vi "Teleop.vi"(10 "Match Info":T1={"Autonomous Elapsed Seconds"=0.0, "TeleOp Elapsed Seconds"=0.0, "Disabled Elapsed Seconds"=0.0, "Visited Autonomous"=FALSE, "Visited TeleOp"=FALSE, "Visited Disabled"=FALSE, "Autonomous Settings"={"Autonomous Style"=enum."Independent", "VI Refnum"=refnum}}, 11 "Call Context":T2) -> ()   [LabVIEW 2018]
doc: "This VI is called for each TeleOp packet received from the DS where the robot is not disabled. It is often used to read from the joysticks and update I/O or to update setpoints for timed control loops. It should complete and return within 20 milliseconds or it may miss DS packets."
uses:
  <vilib>/Rock Robotics/WPI/DriverStation/WPI_DriverStationDerivedRobotMode.ctl
  <vilib>/Rock Robotics/WPI/DriverStation/WPI_DriverStationMatch Info.ctl
  <vilib>/Rock Robotics/WPI/Solenoid/WPI_SolenoidValue.ctl
  <vilib>/Rock Robotics/WPI/ThirdParty/Phoenix-LabVIEW/Motor Controller/Controls/CTRE_Phoenix_MotorControl_ControlMode.ctl
  <vilib>/Rock Robotics/WPI/Utilities/WPI_GetSetVariantRefNum.vi
  Robot Global Data.vi
  <vilib>/Rock Robotics/Network Tables/NT Write Boolean Array.vi
  <vilib>/Rock Robotics/Network Tables/NT Write Numeric Array.vi
  <vilib>/Rock Robotics/Network Tables/NT Read Boolean.vi
  <vilib>/Rock Robotics/Network Tables/NT Read Number.vi
  <vilib>/Rock Robotics/WPI/Solenoid/WPI_SolenoidSetEnum.vi
panel:
  out "Sample Slider 0":dbl(slide) scale=0.0..5.0
  out "Sample Boolean 1":bool
  out "Sample Boolean 0":bool
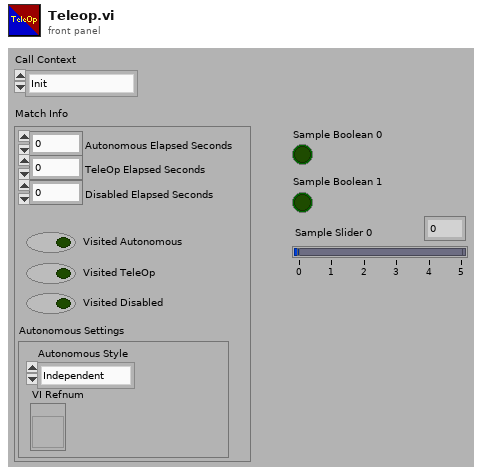
[diagram p1: front panel]
types:
  T1 = typedef "WPI_DriverStationMatch Info.ctl" = cluster{"Autonomous Elapsed Seconds":dbl, "TeleOp Elapsed Seconds":dbl, "Disabled Elapsed Seconds":dbl, "Visited Autonomous":bool, "Visited TeleOp":bool, "Visited Disabled":bool, "Autonomous Settings":cluster{"Autonomous Style":enum16{"Iterative", "Independent"}, "VI Refnum":refnum<vi>}}
  T2 = typedef "WPI_DriverStationDerivedRobotMode.ctl" = enum16{"Init", "Execute", "Stop"}
  T3 = typedef "CTRE_Phoenix_MotorControl_ControlMode.ctl" = u16
  T4 = typedef "WPI_SolenoidValue.ctl" = enum16{"Off", "On", "Forward", "Reverse"}
  T5 = typedef "WPI_JoystickDevRef.ctl" = cluster{"Device":T6}
  T6 = typedef "WPI_JoystickDeviceEnum.ctl" = enum16{"USB 0", "USB 1", "USB 2", "USB 3", "USB 4", "USB 5"}
  T7 = typedef "WPI_RobotDriveDevRef.ctl" = cluster{"DevStatus":errorcluster, "Motors[]":T8[], "Square Inputs":bool, "Max Output":dbl}
  T8 = typedef "WPI_MotorControlDeviceRef.ctl" = cluster{"DeviceStatus":errorcluster, "Type":T9, "PWM":cluster{"PWM Channel":T10, "DeadBand":T11}, "CAN":cluster{"Device Number":u8, "SetOutput VI Ref":variant, "GetOutput VI Ref":variant, "Enable VI Ref":variant, "Disable VI Ref":variant, "Data":variant}, "Invert":bool, "DIO PWM":cluster{"PWM \"Enable\" Channel":T10, "DIOChannel":T12, "PWM Rate":dbl}}
  T9 = typedef "WPI_MotorControlType.ctl" = enum16{"PWM", "CAN", "DIO PWM"}
  T10 = typedef "FPGA_DIOPWMChannel.ctl" = enum8{"PWM 0", "PWM 1", "PWM 2", "PWM 3", "PWM 4", "PWM 5", "PWM 6", "PWM 7", "PWM 8", "PWM 9", "PWM MXP 0", "PWM MXP 1", "PWM MXP 2", "PWM MXP 3", "PWM MXP 4", "PWM MXP 5", "PWM MXP 6", "PWM MXP 7", "PWM MXP 8", "PWM MXP 9", "Invalid"}
  T11 = typedef "WPI_PWMDeadband.ctl" = cluster{"Name":string, "maxPositivePwm":i32, "minPositivePwm":i32, "centerPwm":i32, "maxNegativePwm":i32, "minNegativePwm":i32, "angularRange":u16}
  T12 = typedef "FPGA_DIOChannel.ctl" = enum8{"DIO 0", "DIO 1", "DIO 2", "DIO 3", "DIO 4", "DIO 5", "DIO 6", "DIO 7", "DIO 8", "DIO 9", "DIO MXP 0", "DIO MXP 1", "DIO MXP 2", "DIO MXP 3", "DIO MXP 4", "DIO MXP 5", "DIO MXP 6", "DIO MXP 7", "DIO MXP 8", "DIO MXP 9", "DIO MXP 10", "DIO MXP 11", "DIO MXP 12", "DIO MXP 13", "DIO MXP 14", "DIO MXP 15", "SPI Port CS1", "SPI Port CS2", "SPI Port CS3", "SPI Port MISO", "SPI Port MOSI", "Invalid"}
  T13 = cluster{"Buttons[0]":bool, "Buttons[1]":bool, "Buttons[2]":bool, "Buttons[3]":bool, "Buttons[4]":bool, "Buttons[5]":bool, "Buttons[6]":bool, "Buttons[7]":bool, "Buttons[8]":bool, "Buttons[9]":bool, "Buttons[10]":bool}
  T14 = typedef "WPI_SolenoidDevRef.ctl" = cluster{"DevStatus":errorcluster, "Pneumatics Control Module":u8, "Forward Solenoid Channel":T15, "Reverse Solenoid Channel":T15}
  T15 = typedef "WPI_SolenoidChannel.ctl" = enum8{"Solenoid 0", "Solenoid 1", "Solenoid 2", "Solenoid 3", "Solenoid 4", "Solenoid 5", "Solenoid 6", "Solenoid 7", "Invalid"}
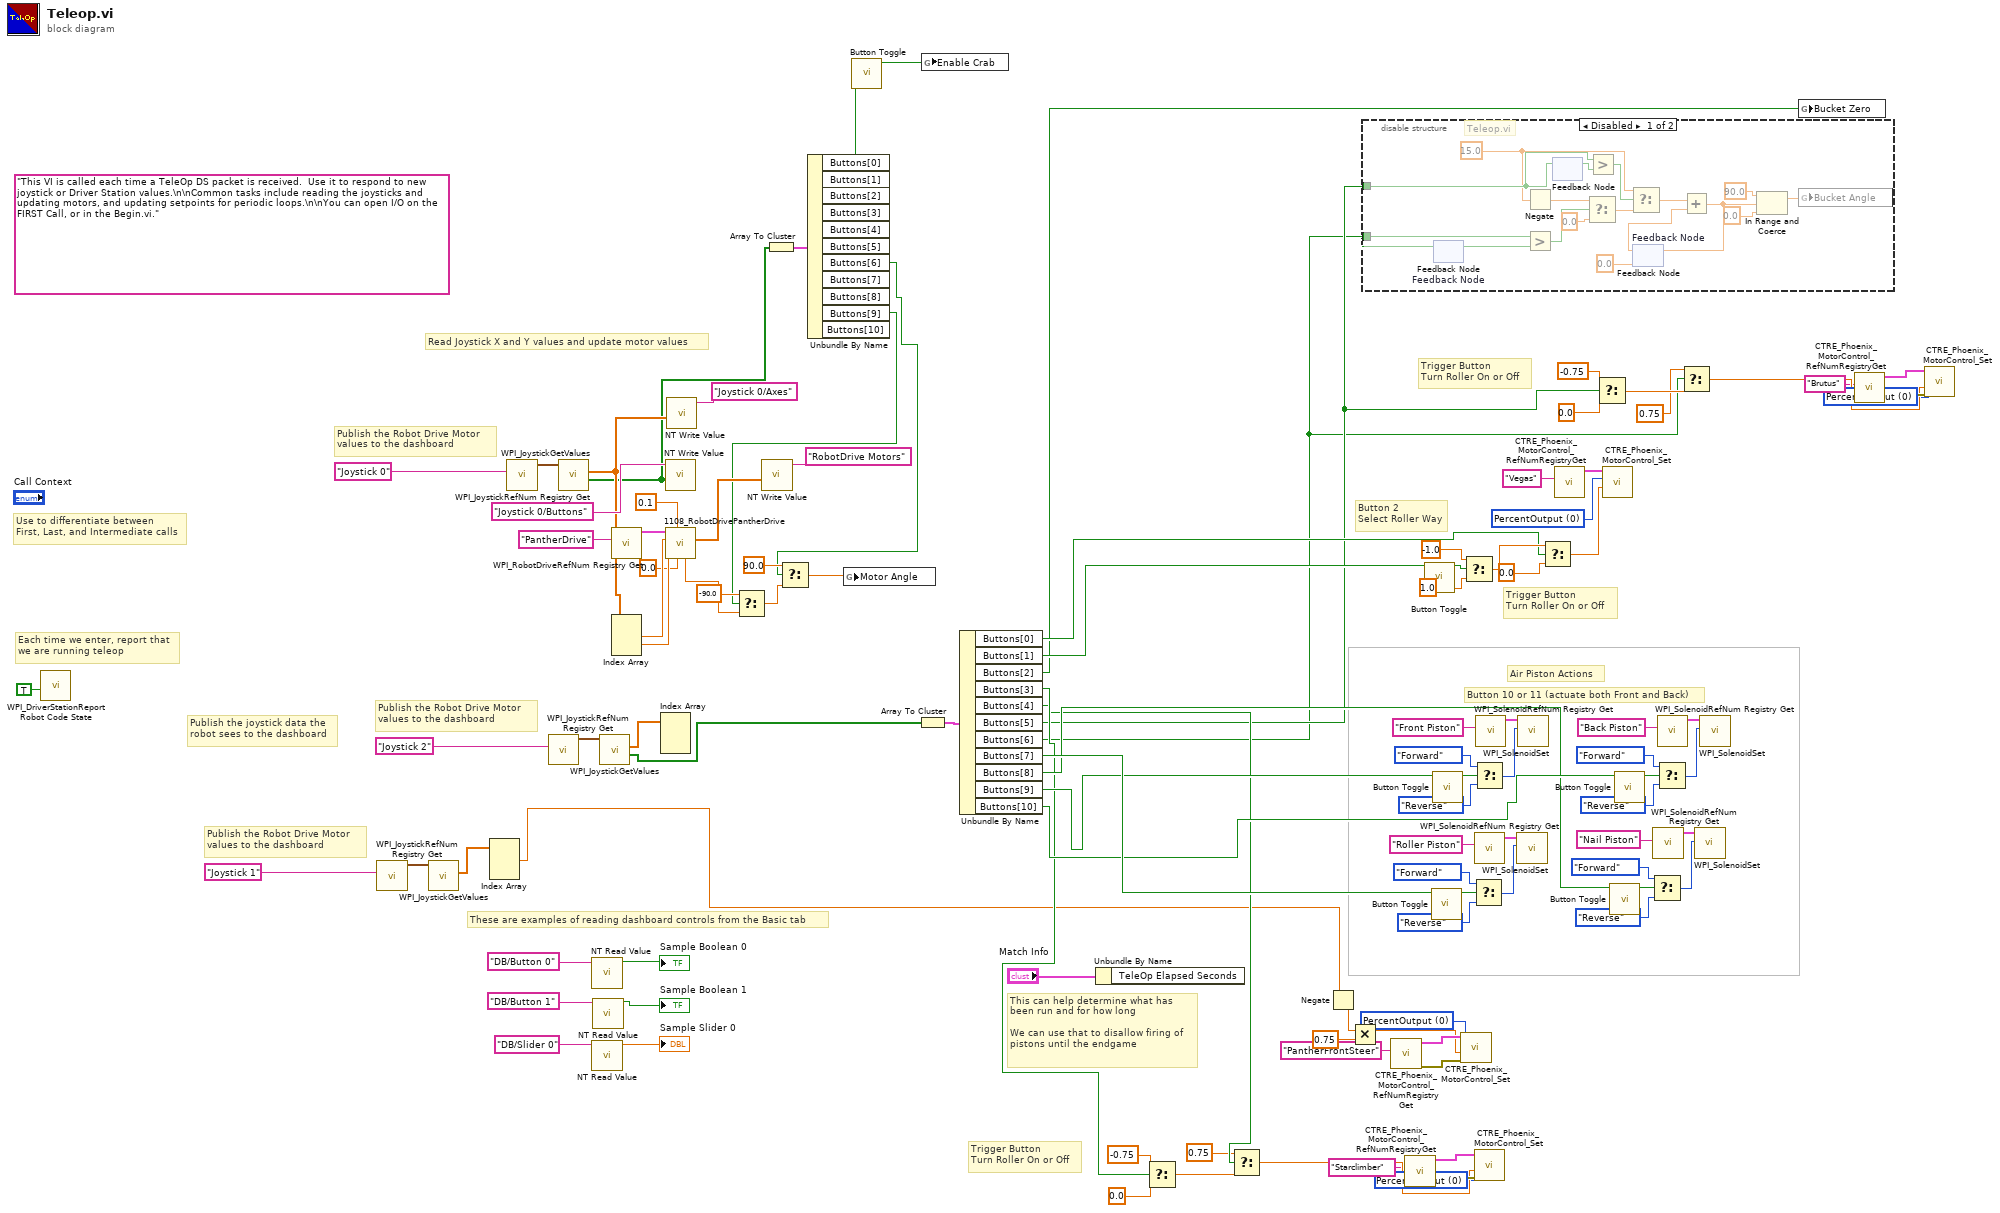
[diagram p0: block diagram]
diagram:
  w23 = T3 0 items=["PercentOutput"=0, "Position"=1, "Velocity"=2, "Current"=3, "Follower"=5, "MotionProfile"=6, "MotionMagic"=7, "MotionProfileArc"=10, "Disabled"=15] ("Control Mode")
  w32 = T3 0 items=["PercentOutput"=0, "Position"=1, "Velocity"=2, "Current"=3, "Follower"=5, "MotionProfile"=6, "MotionMagic"=7, "MotionProfileArc"=10, "Disabled"=15] ("Control Mode")
  w43 = T3 0 items=["PercentOutput"=0, "Position"=1, "Velocity"=2, "Current"=3, "Follower"=5, "MotionProfile"=6, "MotionMagic"=7, "MotionProfileArc"=10, "Disabled"=15] ("Control Mode")
  w59 = T3 0 items=["PercentOutput"=0, "Position"=1, "Velocity"=2, "Current"=3, "Follower"=5, "MotionProfile"=6, "MotionMagic"=7, "MotionProfileArc"=10, "Disabled"=15] ("Control Mode")
  (unwired) "This VI is called each time a TeleOp DS packet is received.  Use it to respond to new joystick or Driver Station values.\n\nCommon tasks include reading the joysticks and updating motors, and updating setpoints for periodic loops.\n\nYou can open I/O on the FIRST Call, or in the Begin.vi."
  # "Publish the Robot Drive Motor\nvalues to the dashboard"
  # "Trigger Button\nTurn Roller On or Off"
  # "Trigger Button\nTurn Roller On or Off"
  # "Button 2\nSelect Roller Way"
  # "Trigger Button\nTurn Roller On or Off"
  # "Button 10 or 11 (actuate both Front and Back)"
  # "Air Piston Actions"
  # "Publish the Robot Drive Motor\nvalues to the dashboard"
  # "These are examples of reading dashboard controls from the Basic tab"
  # "Publish the Robot Drive Motor\nvalues to the dashboard"
  # "Publish the joystick data the\nrobot sees to the dashboard"
  # "Each time we enter, report that\nwe are running teleop"
  # "Use to differentiate between\nFirst, Last, and Intermediate calls"
  # "This can help determine what has\nbeen run and for how long\n\nWe can use that to disallow firing of\npistons until the endgame"
  # "Read Joystick X and Y values and update motor values"
  n1 = call <vilib>:"WPI_DriverStationReport Robot Code State.vi"("TeleOp"=TRUE ("Autonomous")) -> ()  [unwired: 10 in, 1 out]
  n2 = call <vilib>:"WPI_JoystickRefNum Registry Get.vi"("refnum name"="Joystick 1") -> ("JoystickDevRef"=w15:T5)  [unwired: 1 in, 9 out]
  n3 = call <vilib>:"WPI_JoystickGetValues.vi"("JoystickDevRef"=w15) -> ("Axes"=w14:dbl[])  [unwired: 6 in, 4 out]
  n4 = Index Array(array=w14) -> (element #1=w13:dbl)  [unwired: 3 in, 2 out]
  n5 = call <vilib>:"WPI_JoystickRefNum Registry Get.vi"("refnum name"="Joystick 0") -> ("JoystickDevRef"=w107:T5)  [unwired: 1 in, 9 out]
  n6 = call <vilib>:"WPI_JoystickRefNum Registry Get.vi"("refnum name"="Joystick 2") -> ("JoystickDevRef"=w90:T5)  [unwired: 1 in, 9 out]
  n7 = call <vilib>:"WPI_JoystickGetValues.vi"("JoystickDevRef"=w107) -> ("Buttons"=w11:bool[], "Axes"=w103:dbl[])  [unwired: 6 in, 3 out]
  n8 = call-poly <vilib>:"NT Read Value.vi"("Name"="DB/Button 0" ("refnum name")) -> ("Boolean"=→"Sample Boolean 0":bool)  [unwired: 9 in, 1 out]
  n9 = call-poly <vilib>:"NT Read Value.vi"("Name"="DB/Slider 0" ("refnum name")) -> ("Numeric"=→"Sample Slider 0":dbl)  [unwired: 9 in, 1 out]
  n10 = call-poly <vilib>:"NT Read Value.vi"("Name"="DB/Button 1" ("refnum name")) -> ("Boolean"=→"Sample Boolean 1":bool)  [unwired: 9 in, 1 out]
  n11 = call <vilib>:"WPI_JoystickGetValues.vi"("JoystickDevRef"=w90) -> ("Buttons"=w87:bool[], "Axes"=w89:dbl[])  [unwired: 6 in, 3 out]
  n12 = call <vilib>:"WPI_RobotDriveRefNum Registry Get.vi"("refnum name"="PantherDrive") -> ("RobotDriveDevRef"=w94:T7)  [unwired: 1 in, 9 out]
  n13 = Index Array(array=w103) -> (element #1=w93:dbl, element #2=w92:dbl)  [unwired: 3 in, 1 out]
  n14 = Index Array(array=w89) -> ()  [unwired: 3 in, 3 out]
  n15 = call-poly <vilib>:"NT Write Value.vi"("Boolean Array"=w11, "Name"="Joystick 0/Buttons") -> ()  [unwired: 9 in, 1 out]
  n16 = call "1108_RobotDrivePantherDrive.vi"("x-spin"=0.0, "Deadband"=0.1, "y"=w92, "x"=w93, "RobotDriveDevRef"=w94) -> ("Motor Values"=w95:dbl[], "Motor angle"=w8:dbl)  [unwired: 3 in, 2 out]
  n17 = call-poly <vilib>:"NT Write Value.vi"("Numeric Array"=w103, "Name"="Joystick 0/Axes") -> ()  [unwired: 9 in, 1 out]
  n18 = call-poly <vilib>:"NT Write Value.vi"("Numeric Array"=w95, "Name"="RobotDrive Motors") -> ()  [unwired: 9 in, 1 out]
  n19 = Array To Cluster(array=w11) -> (cluster=w12:T13)
  n20 = Unbundle By Name(w12) -> ("Buttons[0]"=w10:bool, "Buttons[6]"=w3:bool, "Buttons[9]"=w4:bool)  [unwired: 8 out]
  n21 = Select(t=-90.0, s=w4, f=w8) -> (s? t:f=w7:dbl)
  n22 = Select(t=90.0, s=w3, f=w7) -> (s? t:f=w2:dbl)
  n23 = global write "Robot Global Data.vi" "Motor Angle"(w2) -> ()
  n24 = call "Button Toggle.vi"("Button Input"=w10) -> ("Toggled Output"=w9:bool)  [unwired: 10 in]
  n25 = Array To Cluster(array=w87) -> (cluster=w88:T13)
  n26 = global write "Robot Global Data.vi" "Enable Crab"(w9) -> ()
  n27 = Unbundle By Name(w88) -> ("Buttons[0]"=w51:bool, "Buttons[1]"=w55:bool, "Buttons[2]"=w50:bool, "Buttons[3]"=w36:bool, "Buttons[4]"=w35:bool, "Buttons[5]"=w20:bool, "Buttons[6]"=w19:bool, "Buttons[7]"=w52:bool, "Buttons[8]"=w42:bool, "Buttons[9]"=w48:bool, "Buttons[10]"=w49:bool)
  n28 = Unbundle By Name("Match Info") -> ()  [unwired: 1 out]
  n29 = Select(t=-0.75, s=w36, f=0.0) -> (s? t:f=w31:dbl)
  n30 = Select(t=0.75 ("f"), s=w35, f=w31) -> (s? t:f=w37:dbl)
  n31 = Negate(x=w13) -> (-x=w17:dbl)
  n32 = Multiply(x=w17, y=0.75) -> (x*y=w45:dbl)
  n33 = disable-structure shown="Disabled" {
    disable-tunnel: w19 -> [w118 _]
    disable-tunnel: w20 -> [w117 _]
    frame Disabled {
      w115 = 15.0 ("t")
      # "Teleop.vi"
      n34 = feedback #1 "Feedback Node"() -> (w126:bool)  [unwired: 1 in]
      n35 = feedback-in #1(w118) -> ()
      n36 = Negate(x=w115) -> (-x=w114:dbl)
      n37 = Greater?(x=w118, y=w126) -> (0:w125:bool)
      n38 = feedback #2() -> (w127:bool)  [unwired: 1 in]
      n39 = feedback-in #2(w117) -> ()
      n40 = Select(t=w114, s=w125, f=0.0) -> (s? t:f=w123:dbl)
      n41 = Greater?(x=w117, y=w127) -> (0:w122:bool)
      n42 = Select(t=w115, s=w122, f=w123) -> (s? t:f=w121:dbl)
      n43 = feedback #3 "Feedback Node"(0.0) -> (w120:dbl)
      n44 = Add(x=w121, y=w120) -> (x+y=w116:dbl)
      n45 = feedback-in #3(w116) -> ()
      n46 = In Range and Coerce(upper limit=90.0, x=w116, lower limit=0.0) -> (coerced(x)=w111:dbl)  [unwired: 1 out]
      n47 = global write "Robot Global Data.vi" "Bucket Angle"(w111) -> ()
    }
    frame Enabled {
    }
  }
  n48 = call <vilib>:"CTRE_Phoenix_MotorControl_RefNumRegistryGet.vi"("refnum name"="PantherFrontSteer") -> ("error out"=w47:errorcluster, "PhoenixMotorControlDevRef"=w46:T8)  [unwired: 9 in]
  n49 = call <vilib>:"CTRE_Phoenix_MotorControl_RefNumRegistryGet.vi"("refnum name"="Starclimber") -> ("error out"=w41:errorcluster, "PhoenixMotorControlDevRef"=w40:T8)  [unwired: 9 in]
  n50 = call "Button Toggle.vi"("Button Input"=w55) -> ("Toggled Output"=w62:bool)  [unwired: 10 in]
  n51 = call "Button Toggle.vi"("Button Input"=w52) -> ("Toggled Output"=w74:bool)  [unwired: 10 in]
  n52 = call "Button Toggle.vi"("Button Input"=w48) -> ("Toggled Output"=w86:bool)  [unwired: 10 in]
  n53 = call <vilib>:"CTRE_Phoenix_MotorControl_Set.vi"("error in (no error)"=w47, "Output"=w45, "Control Mode"=w43, "PhoenixMotorControlDevRef"=w46) -> ()  [unwired: 6 in, 2 out]
  n54 = Select(t=-1.0, s=w62, f=1.0) -> (s? t:f=w56:dbl)
  n55 = Select(t=WPI_SolenoidValue."Forward" ("Value"), s=w74, f=WPI_SolenoidValue."Reverse" ("Value")) -> (s? t:f=w73:T4)
  n56 = Select(t=WPI_SolenoidValue."Forward" ("Value"), s=w86, f=WPI_SolenoidValue."Reverse" ("Value")) -> (s? t:f=w85:T4)
  n57 = call <vilib>:"WPI_SolenoidRefNum Registry Get.vi"("refnum name"="Roller Piston") -> ("SolenoidDevRef"=w70:T14)  [unwired: 9 in, 1 out]
  n58 = call <vilib>:"CTRE_Phoenix_MotorControl_Set.vi"("error in (no error)"=w41, "Output"=w37, "Control Mode"=w32, "PhoenixMotorControlDevRef"=w40) -> ()  [unwired: 6 in, 2 out]
  n59 = call <vilib>:"WPI_SolenoidRefNum Registry Get.vi"("refnum name"="Front Piston") -> ("SolenoidDevRef"=w82:T14)  [unwired: 9 in, 1 out]
  n60 = call-poly <vilib>:"WPI_SolenoidSet.vi"("Value"=w73, "SolenoidDevRef"=w70) -> ()  [unwired: 8 in, 2 out]
  n61 = call-poly <vilib>:"WPI_SolenoidSet.vi"("Value"=w85, "SolenoidDevRef"=w82) -> ()  [unwired: 8 in, 2 out]
  n62 = Select(t=w56, s=w51, f=0.0) -> (s? t:f=w53:dbl)
  n63 = call <vilib>:"CTRE_Phoenix_MotorControl_RefNumRegistryGet.vi"("refnum name"="Vegas") -> ("PhoenixMotorControlDevRef"=w61:T8)  [unwired: 9 in, 1 out]
  n64 = Select(t=-0.75, s=w20, f=0.0) -> (s? t:f=w22:dbl)
  n65 = call <vilib>:"CTRE_Phoenix_MotorControl_Set.vi"("Output"=w53, "Control Mode"=w59, "PhoenixMotorControlDevRef"=w61) -> ()  [unwired: 7 in, 2 out]
  n66 = call "Button Toggle.vi"("Button Input"=w42) -> ("Toggled Output"=w68:bool)  [unwired: 10 in]
  n67 = call "Button Toggle.vi"("Button Input"=w49) -> ("Toggled Output"=w80:bool)  [unwired: 10 in]
  n68 = Select(t=WPI_SolenoidValue."Forward" ("Value"), s=w68, f=WPI_SolenoidValue."Reverse" ("Value")) -> (s? t:f=w67:T4)
  n69 = call <vilib>:"WPI_SolenoidRefNum Registry Get.vi"("refnum name"="Nail Piston") -> ("SolenoidDevRef"=w64:T14)  [unwired: 9 in, 1 out]
  n70 = Select(t=WPI_SolenoidValue."Forward" ("Value"), s=w80, f=WPI_SolenoidValue."Reverse" ("Value")) -> (s? t:f=w79:T4)
  n71 = call <vilib>:"WPI_SolenoidRefNum Registry Get.vi"("refnum name"="Back Piston") -> ("SolenoidDevRef"=w76:T14)  [unwired: 9 in, 1 out]
  n72 = Select(t=0.75 ("f"), s=w19, f=w22) -> (s? t:f=w25:dbl)
  n73 = call-poly <vilib>:"WPI_SolenoidSet.vi"("Value"=w67, "SolenoidDevRef"=w64) -> ()  [unwired: 8 in, 2 out]
  n74 = call-poly <vilib>:"WPI_SolenoidSet.vi"("Value"=w79, "SolenoidDevRef"=w76) -> ()  [unwired: 8 in, 2 out]
  n75 = global write "Robot Global Data.vi" "Bucket Zero"(w50) -> ()
  n76 = call <vilib>:"CTRE_Phoenix_MotorControl_RefNumRegistryGet.vi"("refnum name"="Brutus") -> ("error out"=w29:errorcluster, "PhoenixMotorControlDevRef"=w28:T8)  [unwired: 9 in]
  n77 = call <vilib>:"CTRE_Phoenix_MotorControl_Set.vi"("error in (no error)"=w29, "Output"=w25, "Control Mode"=w23, "PhoenixMotorControlDevRef"=w28) -> ()  [unwired: 6 in, 2 out]
